vi "close.vi"(8 "error in (no error)":errorcluster, 11 "DevRefnum":u64) -> (0 "error out":errorcluster, 3 "DevRefnum":u64)   [LabVIEW 2013, in "rtlsdr.lvlib"]
doc: "RTLSDR_API int rtlsdr_close(rtlsdr_dev_t *dev);"
uses:
  rtlsdr.lvlib
  rtlsdr.dll
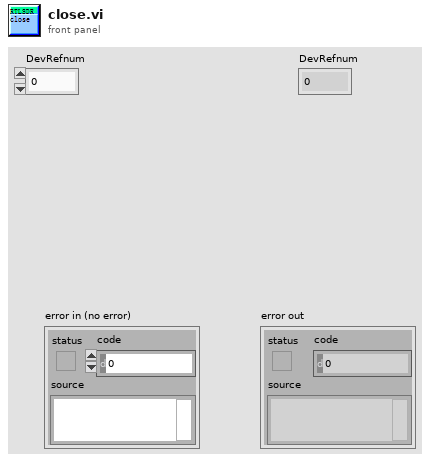
[diagram p1: front panel]
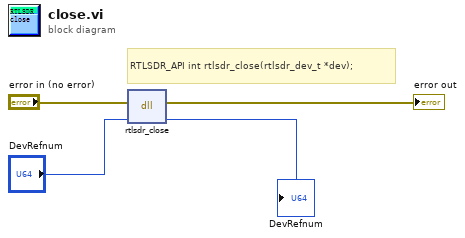
[diagram p0: block diagram]
diagram:
  # "RTLSDR_API int rtlsdr_close(rtlsdr_dev_t *dev);"
  n1 = dll-call lib="PTH1Sabs GCourseCommunication PrinciplesLabWeek10\t第三章rtlsdrrtlsdr.*" fn="rtlsdr_close"(error in="error in (no error)", "dev"="DevRefnum") -> (error out=→"error out":errorcluster, "dev"=→"DevRefnum":u64)  [unwired: 3 in, 1 out]
